vi "Get Logging Directory.vi"(8 "error in":errorcluster, 11 "logging ref":T1=18446744073709551615 format="%.0x") -> (0 "error out":errorcluster, 2 "directory":string, 3 "logging ref out":T1 format="%.0x")   [LabVIEW 2020, in "AIM ARINC 664 Scripting.lvlib"]
uses:
  AIM ARINC 664 Scripting.lvlib
  <vilib>/NI VeriStand/Custom Device API/Custom Device API.lvlib
  <vilib>/NI VeriStand/Custom Device API/Get Item Property (String).vi
  Constants.vi
  <vilib>/NI VeriStand/Custom Device API/Custom Device Item Ref.ctl
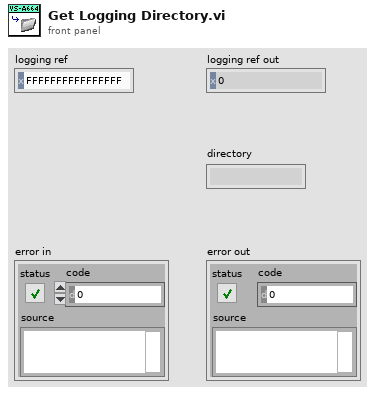
[diagram p1: front panel]
types:
  T1 = typedef "Custom Device API.lvlib/Custom Device Item Ref.ctl" = u64
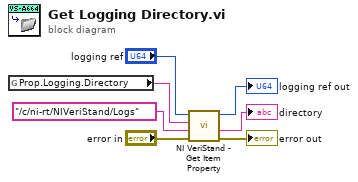
[diagram p0: block diagram]
diagram:
  n1 = global read "Constants.vi" "Prop.Logging.Directory"() -> (w1:string)
  n2 = call-poly <vilib>:"NI VeriStand - Get Item Property.vi"("error in (no error)"="error in", "Default Value"="/c/ni-rt/NIVeriStand/Logs", "Property Name"=w1, "Item Ref in"="logging ref") -> ("error out"=→"error out":errorcluster, "Value"=→"directory":string, "Item Ref out"=→"logging ref out":T1)  [unwired: 4 in, 1 out]
